vi "Select Project.vi"(8 "error in (no error)":errorcluster, 11 "GVIWebProcessorApp in":refnum<class "GVIWebProcessorApp.lvclass">) -> (0 "error out":errorcluster, 2 "Name":string, 3 "GVIWebProcessorApp out":refnum<class "GVIWebProcessorApp.lvclass">)   [LabVIEW 2020, in "PicoG-Processor.lvlib" / "GVIWebProcessorApp.lvclass"]
uses:
  GVIWebProcessorApp.lvclass
  GVIWebProcessorApp.lvclass/GVIWebProcessorApp.ctl
  WebProjectWatcher/WebProjectWatcher.lvclass
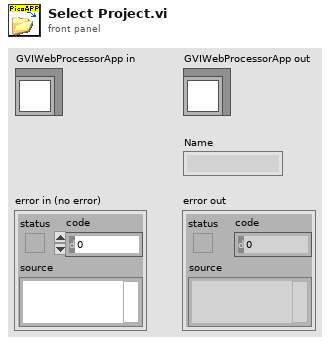
[diagram p1: front panel]
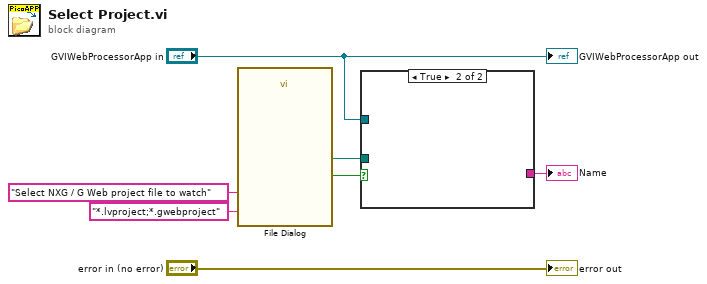
[diagram p0: block diagram]
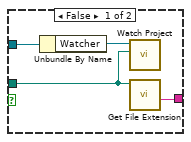
[diagram p2: hidden frame]
diagram:
  n1 = call "File Dialog"("prompt"="Select NXG / G Web project file to watch", "pattern (all files)"="*.lvproject;*.gwebproject") -> ("selected path"=w5:path, "cancelled"=w6:bool)  [unwired: 10 in, 2 out]
  n2 = case shown="True" w6 {
    tunnel: w5 -> [w10 _]
    tunnel: [w9 _] -> w4
    tunnel: "GVIWebProcessorApp in" -> [w8 _]
    frame False {
      n3 = Unbundle By Name(w8) -> ("Watcher"=w11:refnum<class "WebProjectWatcher.lvclass">)
      n4 = call "Watch Project.vi"("Project Path"=w10, "WebProjectWatcher in"=w11) -> ()  [unwired: 8 in, 2 out]
      n5 = call <vilib>:"Get File Extension.vi"("file"=w10) -> ("filename without extension"=w9:string)  [unwired: 6 in, 4 out]
    }
    frame True {
    }
  }
  "Name" <- w4
  "error out" <- "error in (no error)"
  "GVIWebProcessorApp out" <- "GVIWebProcessorApp in"
